vi "SIM Adams manager.vi"(1 "Simulation data":T1={"continuous integrator"=enum."RK 1 (Euler)", "initial time"=0.0, "final time"=6.0, "step size"=0.0, "proposed step size"=0.001, "max step size"=1e-06, "min step size"=0.0, "discrete time step"=0.0, "max step ratio"=3.0, "Diag Eval Stage"=enum."Major Substep", "Substep Index"=0, "Timestep Index"=10.0, "simulation time"=0.0, "current timestep base"=0.1, "proposed step time"=0.0, "absolute tolerance"=0.0, "relative tolerance"=0.0, "step accepted?"=FALSE, "step complete?"=FALSE, "Halt?"=FALSE, "reset integrator?"=FALSE, "machine epsilon"=1.0, "min float"=0.0, "error"={"status"=FALSE, "code"=0, "source"=""}, "Method Order"=0, "Finished Late [i-1]"=FALSE, "Discrete step?"=FALSE, "NaN and Inf check?"=FALSE, "Final Timestep Index"=0.0, "(maj+disc)or(init)?"=FALSE, "Full Solver Reset"=TRUE, "Execution Mode"=enum."Simulate to Completion", "check vector sizes?"=FALSE, "solver handles zc?"=FALSE, "Simulation Registry"={"Current Idx"=0, "Node Tags"=[], "Node Headers"=[], "Node Data"=[], "Cont State data"={"inputs"=[], "outputs"=[], "reset"=[], "lower limits"=[], "upper limits"=[], "limit types"=[], "reset types"=[], "initial conditions"=[], "reset I.C."=[], "limited?"=[], "State Names"=[]}, "DiscreteInfo"={"tick period (sec)"=0.0, "time (ticks)"=0, "fire?"=[], "registry"={"period (sec)"=[], "skew (sec)"=[], "period (tick)"=[], "skew (tick)"=[]}, "discrete \nblocks?"=FALSE, "steps per tick"=0.0, "steps to tick"=0.0, "discrete \ntick?"=FALSE}, "Disc State data"={"Disc States"=[], "State Names"=[]}, "Registry Error"={"Error Block ID"=0, "code"=0}, "ZC Indices"=[]}, "variable step solver?"=FALSE, "First Substep?"=FALSE, "Continuous States?"=FALSE} {"min float" format="%.1e"; "proposed step size" format="%.1e"; "proposed step time" format="%.1e"; "max step ratio" format="%.1e"; "min step size" format="%.1e"; "machine epsilon" format="%.1e"; "discrete time step" format="%.1e"; "max step size" format="%.1e"; "current timestep base" format="%.1e"; "final time" format="%.1e"; "simulation time" format="%.1e"; "relative tolerance" format="%.1e"; "absolute tolerance" format="%.1e"; "Substep Index" format="%.1e"; "step size" format="%.1e"; "initial time" format="%.1e"}) -> (0 "Simulation data out":T1={"continuous integrator"=enum."RK 1 (Euler)", "initial time"=0.0, "final time"=6.0, "step size"=0.0, "proposed step size"=0.001, "max step size"=1e-06, "min step size"=0.0, "discrete time step"=0.0, "max step ratio"=3.0, "Diag Eval Stage"=enum."Major Substep", "Substep Index"=0, "Timestep Index"=10.0, "simulation time"=0.0, "current timestep base"=0.1, "proposed step time"=0.0, "absolute tolerance"=0.0, "relative tolerance"=0.0, "step accepted?"=FALSE, "step complete?"=FALSE, "Halt?"=FALSE, "reset integrator?"=FALSE, "machine epsilon"=1.0, "min float"=0.0, "error"={"status"=FALSE, "code"=0, "source"=""}, "Method Order"=0, "Finished Late [i-1]"=FALSE, "Discrete step?"=FALSE, "NaN and Inf check?"=FALSE, "Final Timestep Index"=0.0, "(maj+disc)or(init)?"=FALSE, "Full Solver Reset"=TRUE, "Execution Mode"=enum."Simulate to Completion", "check vector sizes?"=FALSE, "solver handles zc?"=FALSE, "Simulation Registry"={"Current Idx"=0, "Node Tags"=[], "Node Headers"=[], "Node Data"=[], "Cont State data"={"inputs"=[], "outputs"=[], "reset"=[], "lower limits"=[], "upper limits"=[], "limit types"=[], "reset types"=[], "initial conditions"=[], "reset I.C."=[], "limited?"=[], "State Names"=[]}, "DiscreteInfo"={"tick period (sec)"=0.0, "time (ticks)"=0, "fire?"=[], "registry"={"period (sec)"=[], "skew (sec)"=[], "period (tick)"=[], "skew (tick)"=[]}, "discrete \nblocks?"=FALSE, "steps per tick"=0.0, "steps to tick"=0.0, "discrete \ntick?"=FALSE}, "Disc State data"={"Disc States"=[], "State Names"=[]}, "Registry Error"={"Error Block ID"=0, "code"=0}, "ZC Indices"=[]}, "variable step solver?"=FALSE, "First Substep?"=FALSE, "Continuous States?"=FALSE} {"min float" format="%.1e"; "proposed step size" format="%.1e"; "proposed step time" format="%.1e"; "max step ratio" format="%.1e"; "min step size" format="%.1e"; "machine epsilon" format="%.1e"; "discrete time step" format="%.1e"; "max step size" format="%.1e"; "current timestep base" format="%.1e"; "final time" format="%.1e"; "simulation time" format="%.1e"; "relative tolerance" format="%.1e"; "absolute tolerance" format="%.1e"; "Substep Index" format="%.1e"; "step size" format="%.1e"; "initial time" format="%.1e"})   [LabVIEW 2018]
uses:
  SIM simulation data.ctl
  SIM integration method.ctl
  SIM diagram eval stage.ctl
  SIMSCR Execution Mode.ctl
  SIM Simulation Registry.ctl
  SIM Registry Node Header.ctl
  SIM Registry Node Record.ctl
  SIM trigger type.ctl
  SIM solver state data.ctl
  SIM limit type.ctl
  SIM discrete data.ctl
  SIM Discrete state data.ctl
  SIM Simulation Registry Error.ctl
  SIM Adams stages.ctl
  SIM Adams data.ctl
panel:
  in  "num predictor iterations":i32=1
  in  "Max Order":i32=15
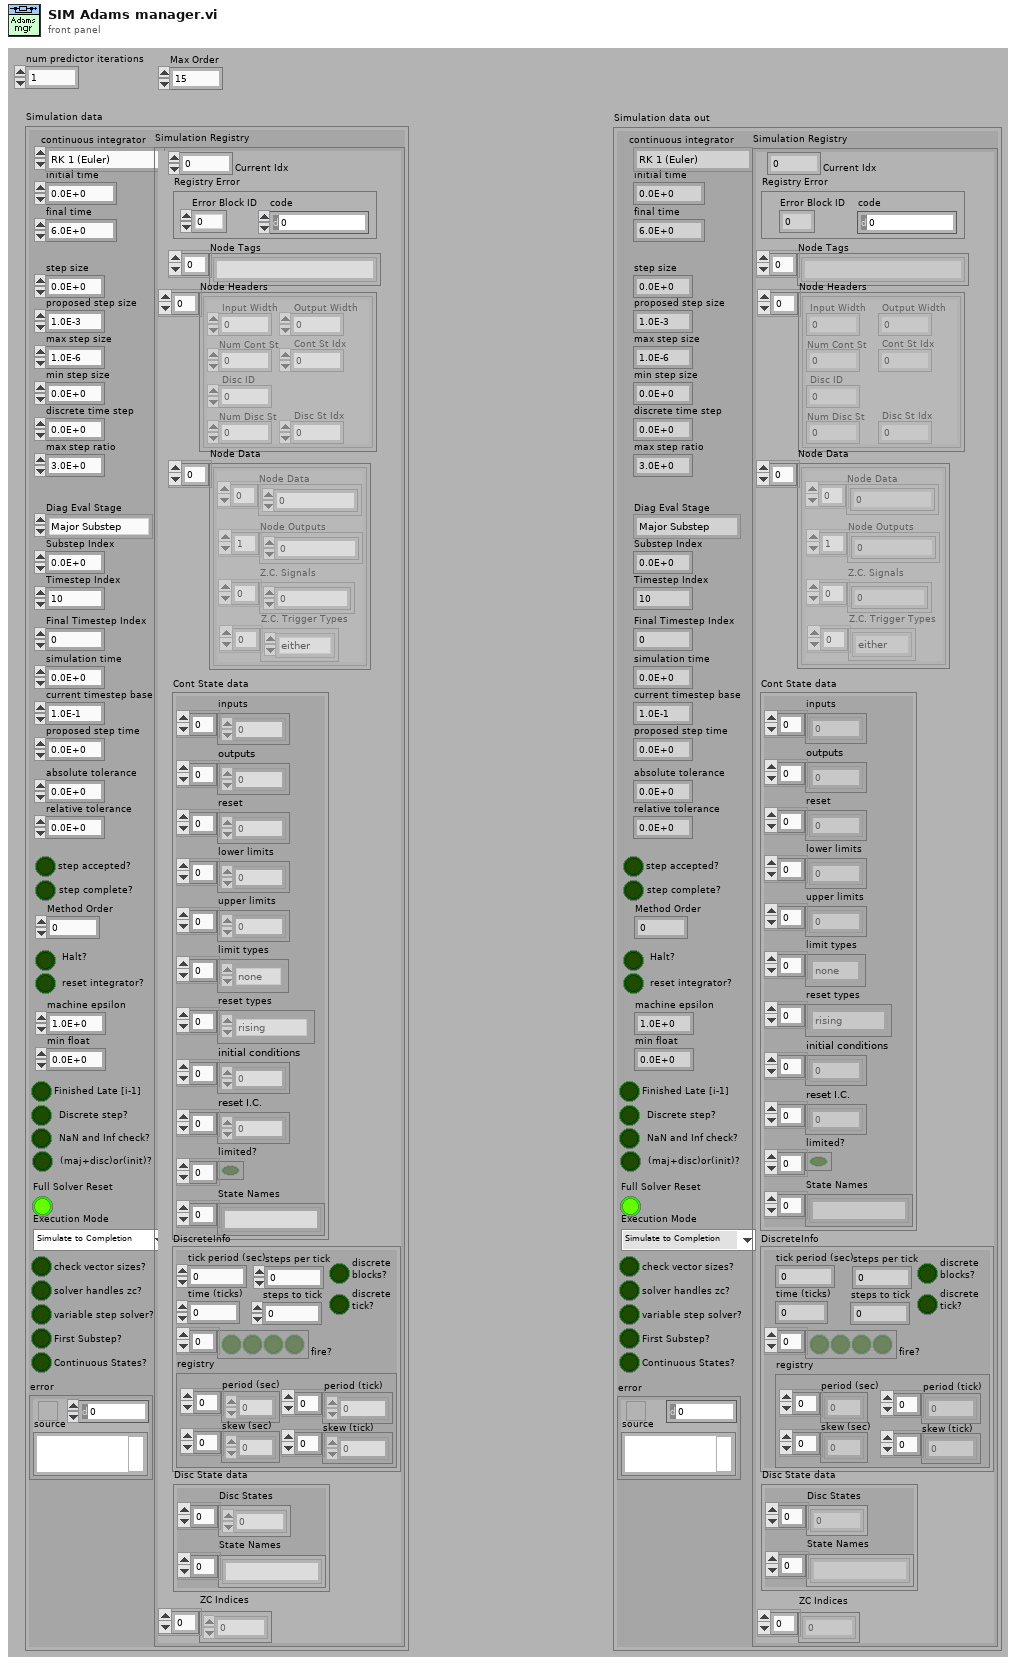
[diagram p1: front panel]
types:
  T1 = typedef "SIM simulation data.ctl" = cluster{"continuous integrator":T2, "initial time":dbl, "final time":dbl, "step size":dbl, "proposed step size":dbl, "max step size":dbl, "min step size":dbl, "discrete time step":dbl, "max step ratio":dbl, "Diag Eval Stage":T3, "Substep Index":i32, "Timestep Index":dbl, "simulation time":dbl, "current timestep base":dbl, "proposed step time":dbl, "absolute tolerance":dbl, "relative tolerance":dbl, "step accepted?":bool, "step complete?":bool, "Halt?":bool, "reset integrator?":bool, "machine epsilon":dbl, "min float":dbl, "error":errorcluster, "Method Order":u32, "Finished Late [i-1]":bool, "Discrete step?":bool, "NaN and Inf check?":bool, "Final Timestep Index":dbl, "(maj+disc)or(init)?":bool, "Full Solver Reset":bool, "Execution Mode":T4, "check vector sizes?":bool, "solver handles zc?":bool, "Simulation Registry":T5, "variable step solver?":bool, "First Substep?":bool, "Continuous States?":bool}
  T2 = typedef "SIM integration method.ctl" = enum16{"RK 1 (Euler)", "Linearizer", "State Query", "Trim Eval", "Adams", "RK 3", "RK 4", "RK 45", "BDF", "RK 2", "RK 23", "Rosenbrock", "Discrete States Only"}
  T3 = typedef "SIM diagram eval stage.ctl" = enum16{"Init", "Minor Substep", "Major Substep", "Final"}
  T4 = typedef "SIMSCR Execution Mode.ctl" = enum16{"Simulate to Completion", "Single Time-Step Simulation (Fixed Step Only)"}
  T5 = typedef "SIM Simulation Registry.ctl" = cluster{"Current Idx":i32, "Node Tags":string[], "Node Headers":T6[], "Node Data":T7[], "Cont State data":T9, "DiscreteInfo":T11, "Disc State data":T12, "Registry Error":T13, "ZC Indices":i32[]}
  T6 = typedef "SIM Registry Node Header.ctl" = cluster{"Input Width":i32, "Disc ID":i32, "Num Cont St":i32, "Cont St Idx":i32, "Num Disc St":i32, "Disc St Idx":i32, "Output Width":i32}
  T7 = typedef "SIM Registry Node Record.ctl" = cluster{"Node Data":dbl[], "Node Outputs":dbl[], "Z.C. Signals":dbl[], "Z.C. Trigger Types":T8[]}
  T8 = typedef "SIM trigger type.ctl" = enum16{"rising", "falling", "either", "none"}
  T9 = typedef "SIM solver state data.ctl" = cluster{"inputs":dbl[], "outputs":dbl[], "reset":dbl[], "lower limits":dbl[], "upper limits":dbl[], "limit types":T10[], "reset types":T8[], "initial conditions":dbl[], "reset I.C.":dbl[], "limited?":bool[], "State Names":string[]}
  T10 = typedef "SIM limit type.ctl" = enum16{"upper", "lower", "both", "none"}
  T11 = typedef "SIM discrete data.ctl" = cluster{"tick period (sec)":dbl, "time (ticks)":i32, "fire?":bool[], "registry":cluster{"period (sec)":dbl[], "skew (sec)":dbl[], "period (tick)":i32[], "skew (tick)":i32[]}, "discrete \nblocks?":bool, "steps per tick":dbl, "steps to tick":dbl, "discrete \ntick?":bool}
  T12 = typedef "SIM Discrete state data.ctl" = cluster{"Disc States":dbl[], "State Names":string[]}
  T13 = typedef "SIM Simulation Registry Error.ctl" = cluster{"Error Block ID":i32, "code":i32}
  T14 = typedef "SIM Adams stages.ctl" = enum16{"Init", "Predict", "Correct", "Eval Error", "Choose StepSize", "Reset BDFs"}
  T15 = typedef "SIM Adams data.ctl" = cluster{"Adams stage":T14, "AB Coeffs":dbl[], "AM Coeffs":dbl[], "BDFs":dbl[][], "last output":dbl[], "zero array":dbl[], "Current Order":i32, "Max Order":i32, "Steps This Order":i32, "Max Err Order":i32, "#Corrections":i32}
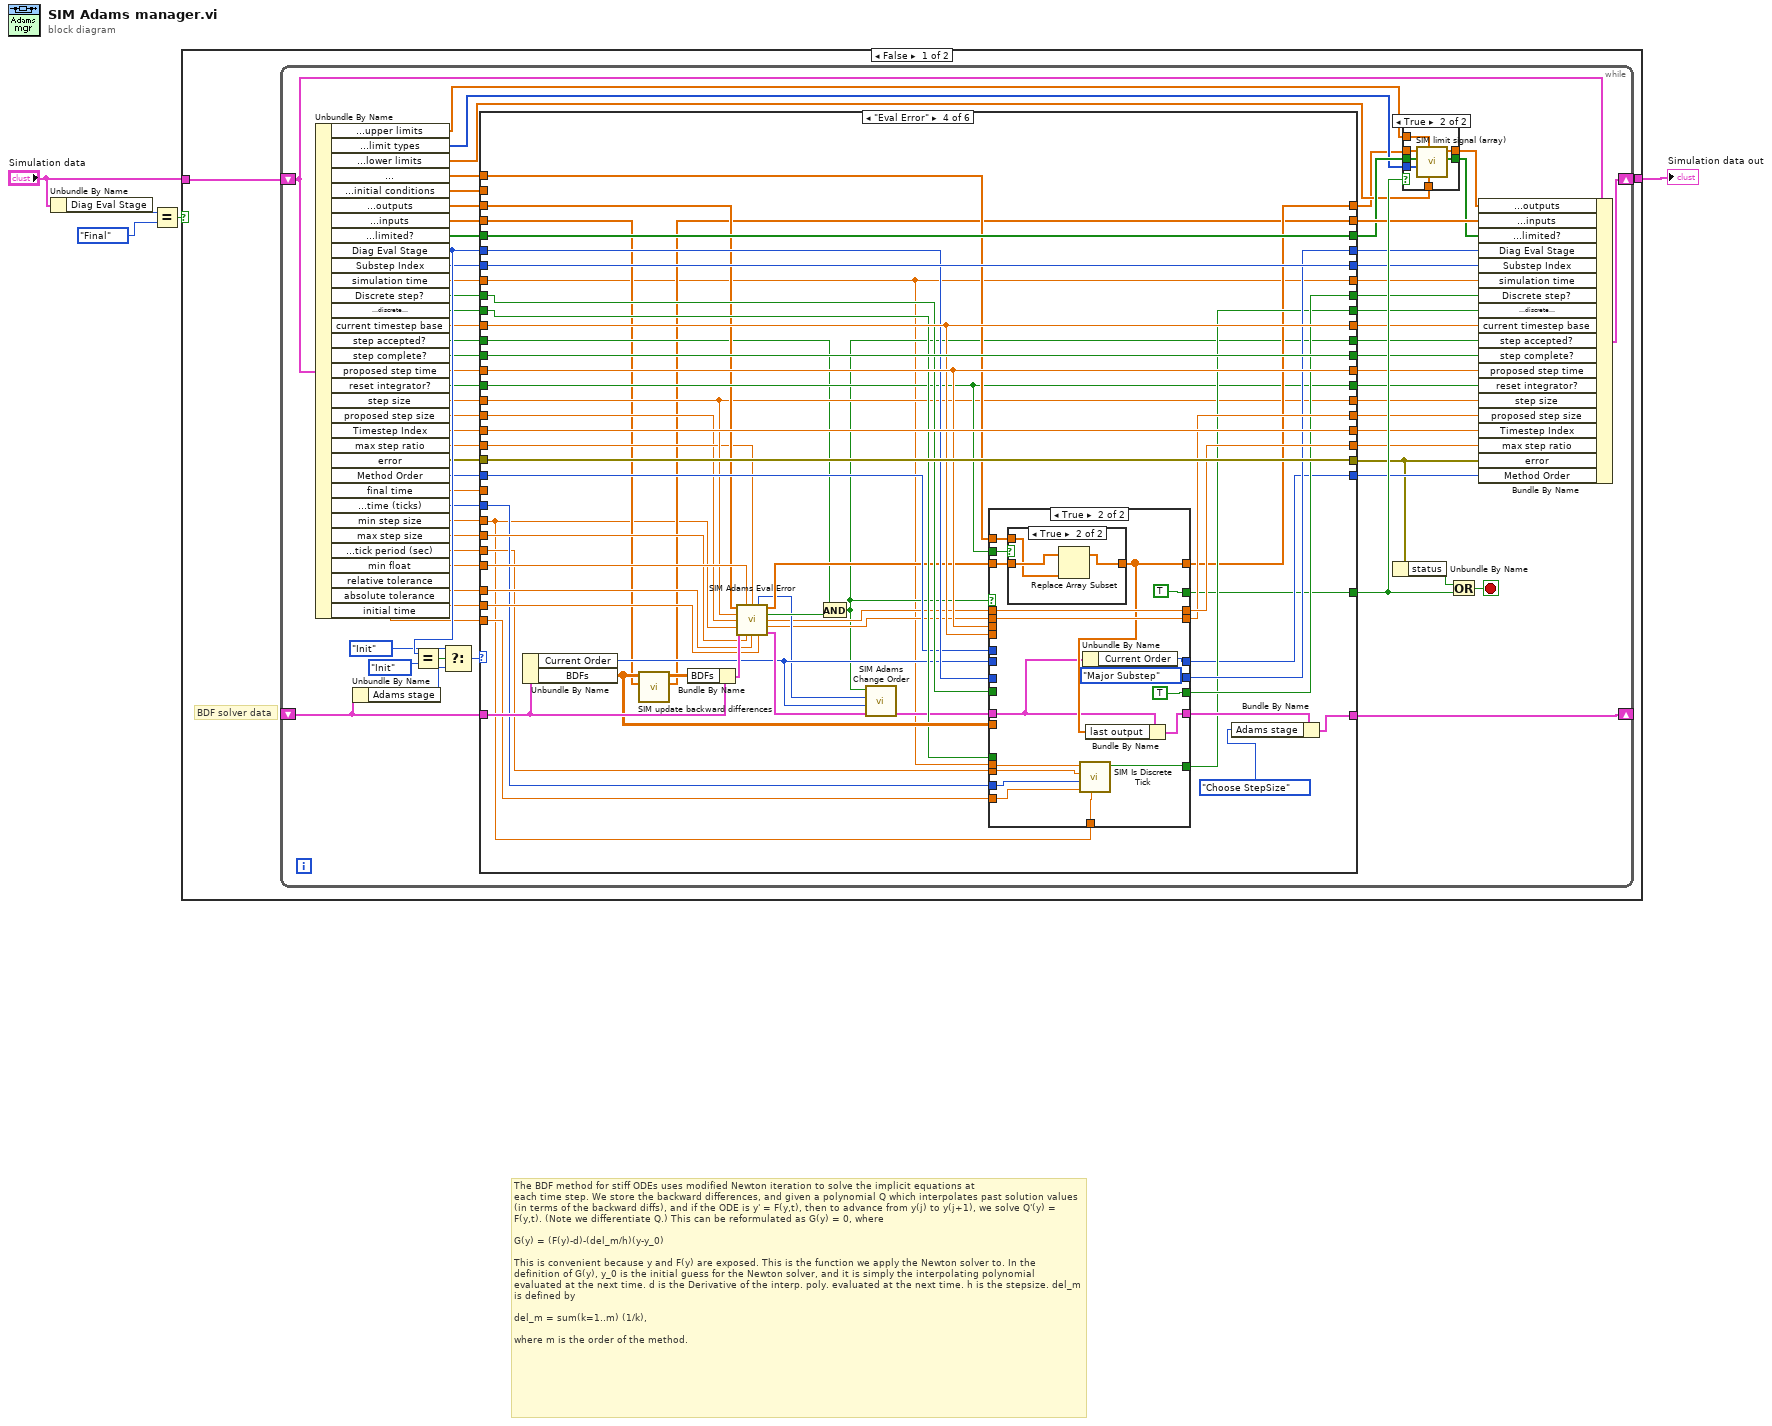
[diagram p0: block diagram]
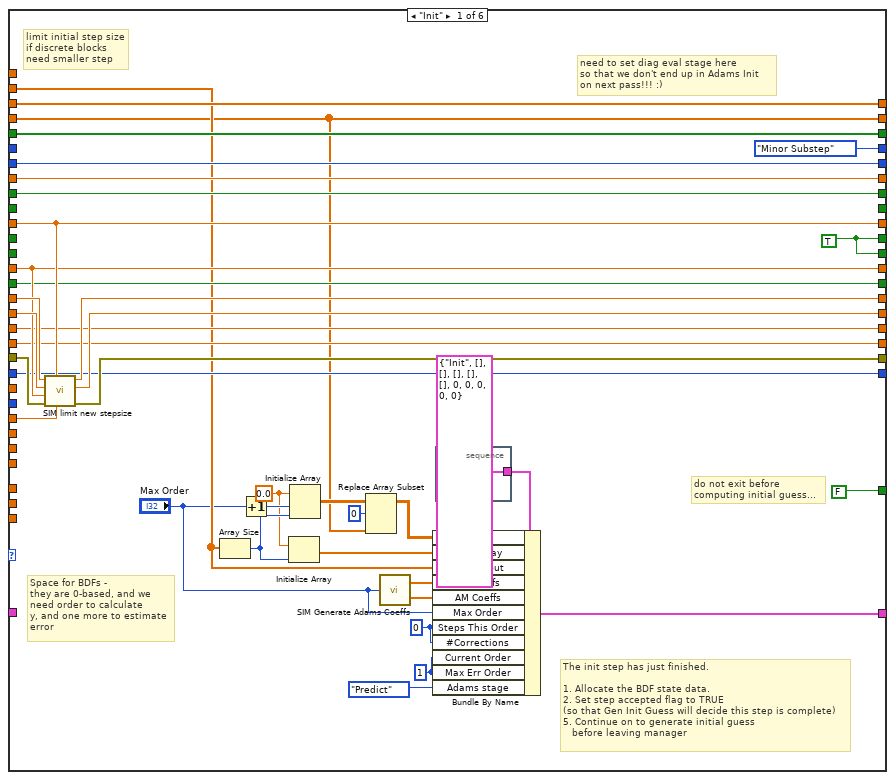
[diagram p3: hidden frame]
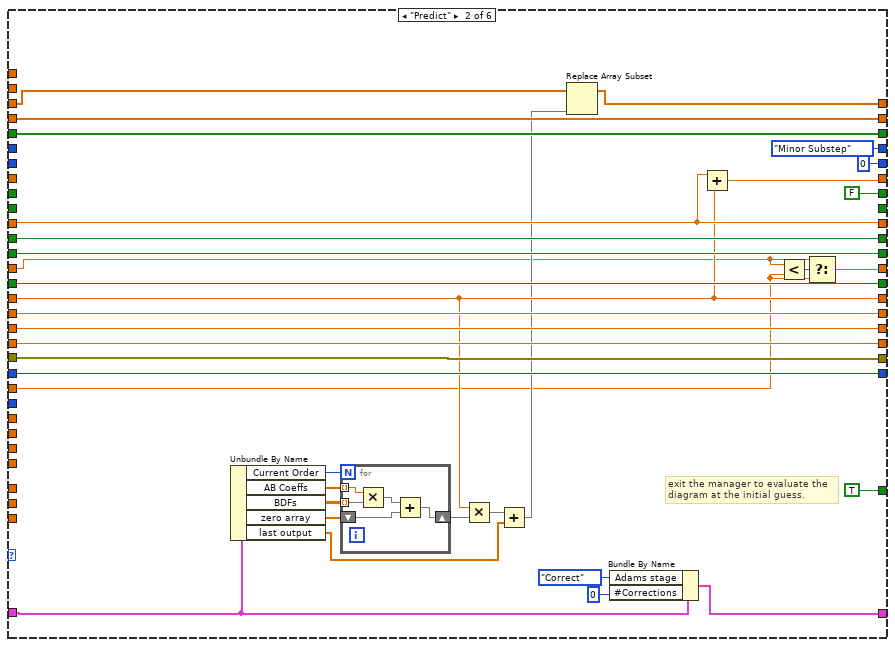
[diagram p4: hidden frame]
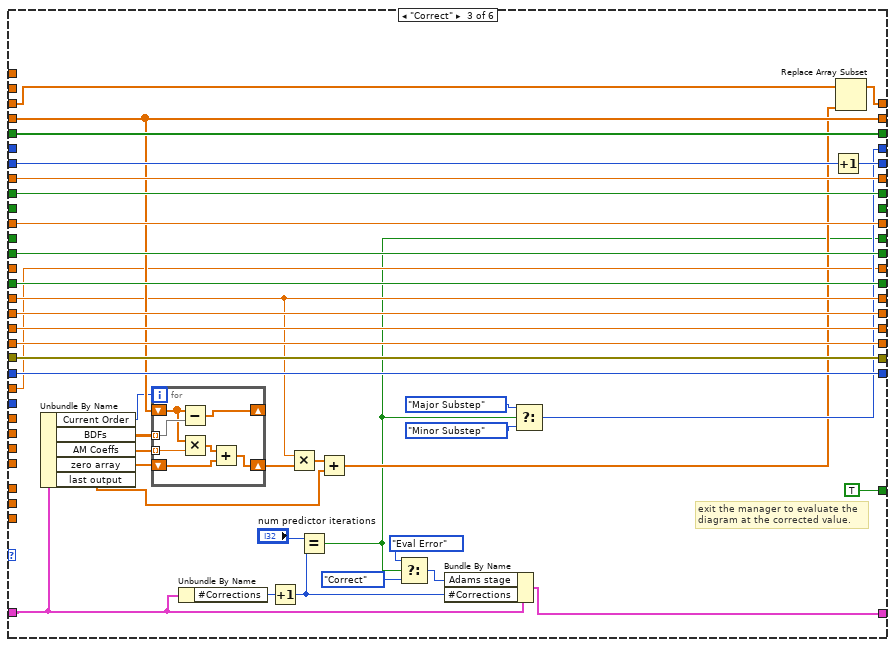
[diagram p5: hidden frame]
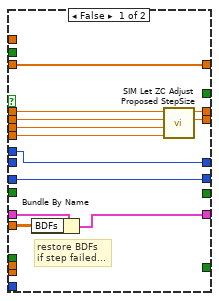
[diagram p6: hidden frame]
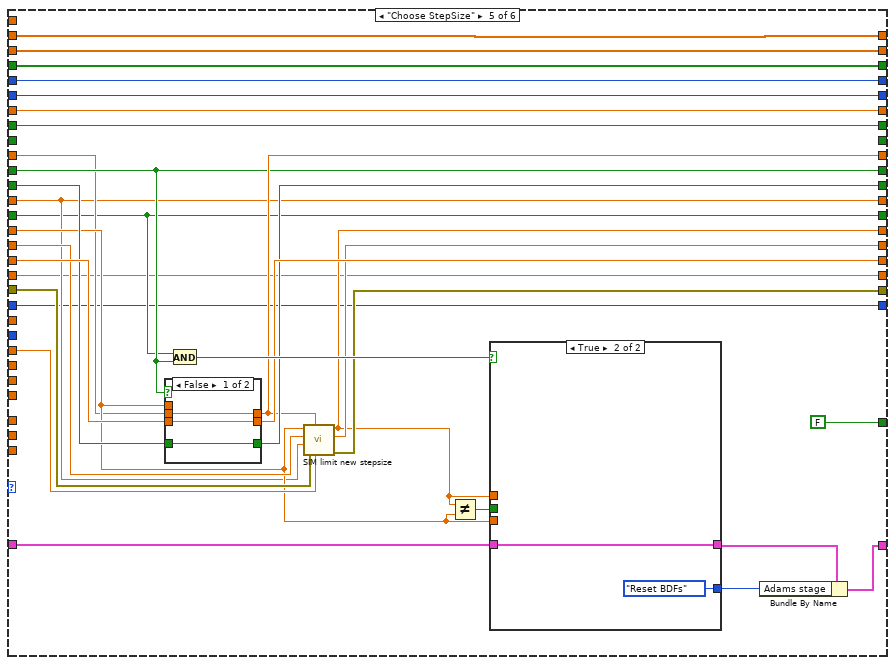
[diagram p8: hidden frame]
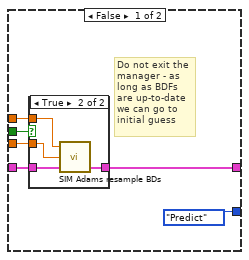
[diagram p9: hidden frame]
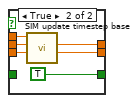
[diagram p11: hidden frame]
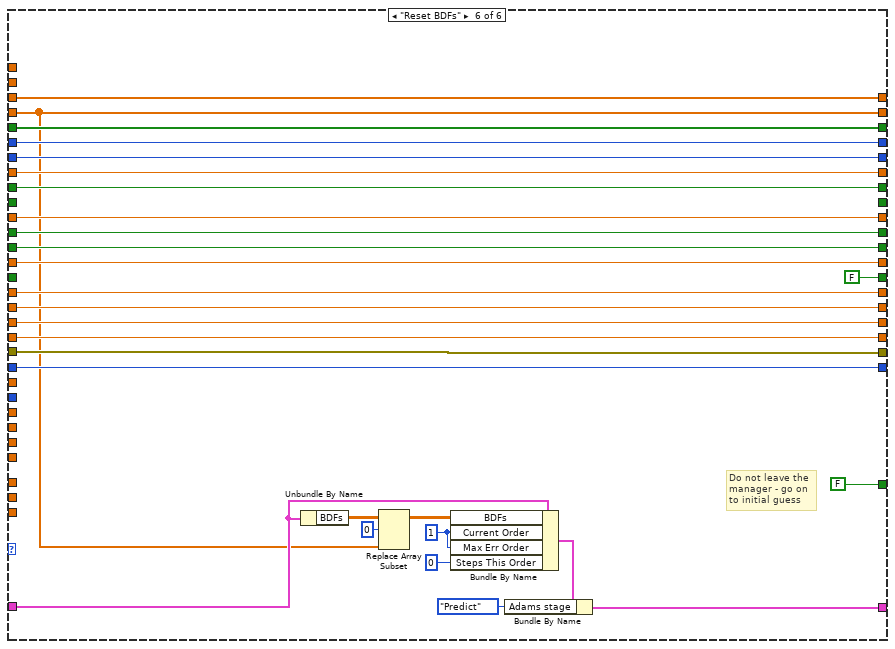
[diagram p12: hidden frame]
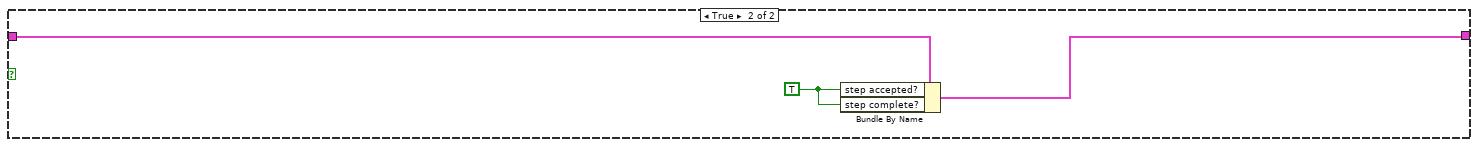
[diagram p13: hidden frame]
diagram:
  # "The BDF method for stiff ODEs uses modified Newton iteration to solve the implicit equations at\neach time step. We store the backward differences, and given a polynomial Q which interpolates past solution values (in terms of the backward diffs), and if the ODE is y' = F(y,t), then to advance from y(j) to y(j+1), we solve Q'(y) = F(y,t). (Note we differentiate Q.) This can be reformulated as G(y) = 0, where \n\nG(y) = (F(y)-d)-(del_m/h)(y-y_0)\n\nThis is convenient because y and F(y) are exposed. This is the function we apply the Newton solver to. In the definition of G(y), y_0 is the initial guess for the Newton solver, and it is simply the interpolating polynomial evaluated at the next time. d is the Derivative of the interp. poly. evaluated at the next time. h is the stepsize. del_m is defined by\n\ndel_m = sum(k=1..m) (1/k),\n\nwhere m is the order of the method."
  n1 = Unbundle By Name("Simulation data") -> ("Diag Eval Stage"=w3:T3)
  n2 = Equal?(x=w3, y=SIM_diagram_eval_stage."Final") -> (x = y?=w1:bool)
  n3 = case shown="False" w1 {
    tunnel: [w7 w378] -> w5
    tunnel: "Simulation data" -> [w6 w377]
    frame False {
      # "BDF solver data"
      n4 = while {
        shift-right: [w33] -> w7
        shift-left: w6 -> [w13]
        shift-right: [w11] -> _
        shift-left: _ -> [w70]
        stop <- w71 stop-if-true
        n5 = Unbundle By Name(w13) -> ("Simulation Registry.Cont State data.upper limits"=w16:dbl[], "Simulation Registry.Cont State data.limit types"=w14:T10[], "Simulation Registry.Cont State data.lower limits"=w15:dbl[], "Simulation Registry.Cont State data.reset I.C."=w24:dbl[], "Simulation Registry.Cont State data.initial conditions"=w28:dbl[], "Simulation Registry.Cont State data.outputs"=w37:dbl[], "Simulation Registry.Cont State data.inputs"=w36:dbl[], "Simulation Registry.Cont State data.limited?"=w30:bool[], "Diag Eval Stage"=w65:T3, "Substep Index"=w63:i32, "simulation time"=w61:dbl, "Discrete step?"=w59:bool, "Simulation Registry.DiscreteInfo.discrete \ntick?"=w57:bool, "current timestep base"=w55:dbl, "step accepted?"=w53:bool, "step complete?"=w51:bool, "proposed step time"=w49:dbl, "reset integrator?"=w47:bool, "step size"=w45:dbl, "proposed step size"=w43:dbl, "Timestep Index"=w41:dbl, "max step ratio"=w39:dbl, "error"=w22:errorcluster, "Method Order"=w21:u32, "final time"=w27:dbl, "Simulation Registry.DiscreteInfo.time (ticks)"=w12:i32, "min step size"=w29:dbl, "max step size"=w25:dbl, "Simulation Registry.DiscreteInfo.tick period (sec)"=w34:dbl, "min float"=w26:dbl, "relative tolerance"=w32:dbl, "absolute tolerance"=w31:dbl, "initial time"=w8:dbl)
        n6 = Unbundle By Name(w70) -> ("Adams stage"=w69:T14)
        n7 = Equal?(x=w65, y=SIM_diagram_eval_stage."Init") -> (x = y?=w67:bool)
        n8 = Select(t=SIM_Adams_stages."Init" ("Adams stage"), s=w67, f=w69) -> (s? t:f=w72:T14)
        n9 = case shown="\"Eval Error\"" w72 {
          tunnel: [FALSE TRUE ("finished?") TRUE ("finished?") w238 FALSE FALSE ("finished?")] -> w66
          tunnel: w70 -> [_ w130 w179 w254 w297 w369]
          tunnel: [SIM_diagram_eval_stage."Minor Substep" ("Diag Eval Stage") SIM_diagram_eval_stage."Minor Substep" ("Diag Eval Stage") w167 w246 w309 w367] -> w64
          tunnel: w65 -> [_ _ _ w245 w309 w367]
          tunnel: [w102 0 ("Substep Index") w199 w256 w308 w366] -> w62
          tunnel: w63 -> [w102 _ w200 w256 w308 w366]
          tunnel: w61 -> [w101 _ w198 w212 w307 w365]
          tunnel: [w101 w145 w198 w212 w307 w365] -> w60
          tunnel: [w100 FALSE ("Discrete step?") w197 w244 w306 w364] -> w58
          tunnel: w59 -> [w100 _ w197 w243 w306 w364]
          tunnel: w57 -> [_ _ _ w241 _ _]
          tunnel: [_ _ _ w242 _ _] -> w56
          tunnel: [w99 w146 w196 w247 w312 w363] -> w54
          tunnel: w55 -> [w99 w146 w196 w247 w304 w363]
          tunnel: [w106 w154 w162 w215 w305 w362] -> w52
          tunnel: w53 -> [_ w154 _ w216 w305 w362]
          tunnel: [w106 w153 w195 w260 w320 w361] -> w50
          tunnel: w51 -> [_ w153 w195 w260 w321 w361]
          tunnel: [w98 w122 w166 w248 w303 w360] -> w48
          tunnel: w49 -> [w98 w123 _ w248 w303 w360]
          tunnel: [w97 w152 w194 w235 w302 FALSE ("reset integrator?")] -> w46
          tunnel: w47 -> [w97 w152 w194 w235 w302 _]
          tunnel: [w107 w135 w171 w230 w314 w359] -> w44
          tunnel: w45 -> [w113 w135 w171 w230 w313 w359]
          tunnel: [w109 w151 w188 w249 w316 w358] -> w42
          tunnel: w43 -> [w112 w151 w188 w219 w319 w358]
          tunnel: [w96 w150 w193 w259 w322 w357] -> w40
          tunnel: w41 -> [w96 w150 w193 w259 w323 w357]
          tunnel: [w95 w149 w187 w250 w300 w356] -> w38
          tunnel: w39 -> [w95 w149 w187 w221 w300 w356]
          tunnel: w37 -> [w104 w128 w164 w233 w296 w350]
          tunnel: w36 -> [w83 w155 w178 w214 w311 w349]
          tunnel: [w104 w126 w163 w237 w296 w350] -> w9
          tunnel: [w83 w155 w178 w213 w311 w349] -> w35
          tunnel: w34 -> [_ _ _ w211 _ _]
          tunnel: w32 -> [_ _ _ w228 _ _]
          tunnel: w31 -> [_ _ _ w227 _ _]
          tunnel: w30 -> [w103 w156 w190 w258 w310 w368]
          tunnel: w22 -> [w111 w148 w192 w257 w318 w355]
          tunnel: w29 -> [w110 _ _ w209 w317 _]
          tunnel: [w108 w148 w192 w257 w315 w355] -> w20
          tunnel: w28 -> [w91 _ _ _ _ _]
          tunnel: [w103 w156 w190 w258 w310 w368] -> w17
          tunnel: w27 -> [_ w124 w166 _ _ _]
          tunnel: w26 -> [_ _ _ w234 _ _]
          tunnel: w25 -> [_ _ _ w229 _ _]
          tunnel: w24 -> [_ _ _ w236 _ _]
          tunnel: [w94 w147 w191 w239 w301 w354] -> w23
          tunnel: w21 -> [w94 w147 w191 w240 w301 w354]
          tunnel: w12 -> [_ _ _ w217 _ _]
          tunnel: [w84 w129 w181 w253 w298 w351] -> w11
          tunnel: w8 -> [_ _ _ w210 _ _]
          frame "Init" {
            w85 = 0 ("Steps This Order")
            w87 = 1 ("Max Order")
            w106 = TRUE ("step complete?")
            w116 = 0.0
            # "need to set diag eval stage here\nso that we don't end up in Adams Init\non next pass!!! :)"
            # "limit initial step size\nif discrete blocks\nneed smaller step"
            # "do not exit before\ncomputing initial guess..."
            # "The init step has just finished.\n\n1. Allocate the BDF state data.\n2. Set step accepted flag to TRUE\n(so that Gen Init Guess will decide this step is complete)\n5. Continue on to generate initial guess\n   before leaving manager"
            # "Space for BDFs - \nthey are 0-based, and we\nneed order to calculate\ny, and one more to estimate\nerror"
            n10 = call "SIM limit new stepsize.vi"("min step size"=w110, "current timestep base"=w99, "error"=w111, "proposed step time"=w98, "proposed step size"=w112, "step size"=w113) -> ("error out"=w108:errorcluster, "proposed step size"=w109:dbl, "step size"=w107:dbl)  [unwired: 3 out]
            n11 = Array Size(array=w91) -> (size(s)=w117:i32)
            n12 = Increment(x="Max Order") -> (x+1=w119:i32)
            n13 = Initialize Array(w116, w117) -> (w92:dbl[])
            n14 = Initialize Array(w116, w119, w117) -> (w114:dbl[][])
            n15 = Replace Array Subset(array=w114, new element=w83, index (row)=0) -> (w118:dbl[][])  [unwired: 1 in]
            n16 = call "SIM Generate Adams Coeffs.vi"("Max Order"="Max Order") -> ("AB Coefficients"=w90:dbl[], "AM Coefficients"=w89:dbl[])
            n17 = stacked-sequence {
              tunnel: [T15 {"Adams stage"=enum."Init", "AB Coeffs"=[], "AM Coeffs"=[], "BDFs"=[], "last output"=[], "zero array"=[], "Current Order"=0, "Max Order"=0, "Steps This Order"=0, "Max Err Order"=0, "#Corrections"=0} ("BDF data")] -> w93
              frame #0 {
              }
            }
            n18 = Bundle By Name(cluster=w93, "BDFs"=w118, "zero array"=w92, "last output"=w91, "AB Coeffs"=w90, "AM Coeffs"=w89, "Max Order"="Max Order", "Steps This Order"=w85, "#Corrections"=w85, "Current Order"=w87, "Max Err Order"=w87, "Adams stage"=SIM_Adams_stages."Predict" ("Enum")) -> (w84:T15)
          }
          frame "Predict" {
            # "exit the manager to evaluate the \ndiagram at the initial guess."
            n19 = Unbundle By Name(w130) -> ("Current Order"=w139:i32, "AB Coeffs"=w138:dbl[], "BDFs"=w142:dbl[][], "zero array"=w141:dbl[], "last output"=w136:dbl[])
            n20 = for {
              N: w139 -> [_]
              shift-right: [w160] -> w140
              shift-left: w141 -> [w161]
              tunnel: w142 -> [w159] mode=indexing
              tunnel: w138 -> [w157] mode=indexing
              n21 = Multiply(x=w157, y=w159) -> (x*y=w158:dbl[])
              n22 = Add(x=w158, y=w161) -> (x+y=w160:dbl[])
            }
            n23 = Multiply(x=w135, y=w140) -> (x*y=w137:dbl[])
            n24 = Add(x=w137, y=w136) -> (x+y=w127:dbl[])
            n25 = Replace Array Subset(array=w128, new element=w127) -> (w126:dbl[])  [unwired: 1 in]
            n26 = Bundle By Name(cluster=w130, "Adams stage"=SIM_Adams_stages."Correct", "#Corrections"=0) -> (w129:T15)
            n27 = Add(x=w146, y=w135) -> (x+y=w145:dbl)
            n28 = Less?(x=w123, y=w124) -> (x < y?=w125:bool)
            n29 = Select(t=w123, s=w125, f=w124) -> (s? t:f=w122:dbl)
          }
          frame "Correct" {
            # "exit the manager to evaluate the \ndiagram at the corrected value."
            n30 = Unbundle By Name(w179) -> ("Current Order"=w176:i32, "BDFs"=w177:dbl[][], "AM Coeffs"=w175:dbl[], "zero array"=w174:dbl[], "last output"=w170:dbl[])
            n31 = for {
              N: w176 -> [_]
              shift-right: [w206] -> w172
              shift-left: w174 -> [w207]
              tunnel: w175 -> [w205] mode=indexing
              tunnel: w177 -> [w203] mode=indexing
              shift-right: [w202] -> _
              shift-left: w178 -> [w201]
              n32 = Subtract(x=w201, y=w203) -> (x-y=w202:dbl[])
              n33 = Multiply(x=w201, y=w205) -> (x*y=w204:dbl[])
              n34 = Add(x=w204, y=w207) -> (x+y=w206:dbl[])
            }
            n35 = Unbundle By Name(w179) -> ("#Corrections"=w186:i32)
            n36 = Increment(x=w186) -> (x+1=w185:i32)
            n37 = Multiply(x=w171, y=w172) -> (x*y=w173:dbl[])
            n38 = Equal?(x="num predictor iterations", y=w185) -> (x = y?=w162:bool)
            n39 = Add(x=w173, y=w170) -> (x+y=w165:dbl[])
            n40 = Select(t=SIM_Adams_stages."Eval Error", s=w162, f=SIM_Adams_stages."Correct" ("Adams stage")) -> (s? t:f=w182:T14)
            n41 = Bundle By Name(cluster=w179, "Adams stage"=w182, "#Corrections"=w185) -> (w181:T15)
            n42 = Select(t=SIM_diagram_eval_stage."Major Substep", s=w162, f=SIM_diagram_eval_stage."Minor Substep" ("Diagram Eval Stage")) -> (s? t:f=w167:T3)
            n43 = Increment(x=w200) -> (x+1=w199:i32)
            n44 = Replace Array Subset(array=w164, new element=w165) -> (w163:dbl[])  [unwired: 1 in]
          }
          frame "Eval Error" {
            n45 = Unbundle By Name(w254) -> ("Current Order"=w223:i32, "BDFs"=w251:dbl[][])
            n46 = call "SIM update backward differences.vi"("New y"=w214, "Backward differences"=w251) -> ("New y out"=w213:dbl[], "New Backward differences"=w255:dbl[][])  [unwired: 8 out]
            n47 = Bundle By Name(cluster=w254, "BDFs"=w255) -> (w231:T15)
            n48 = call "SIM Adams Eval Error.vi"("outputs"=w233, "min float"=w234, "max step ratio"=w221, "step size"=w230, "proposed step size"=w219, "min step size"=w209, "Adams data"=w231, "max step size"=w229, "relative tolerance"=w228, "absolute tolerance"=w227) -> ("proposed new order out"=w222:i32, "outputs out"=w232:dbl[], "step accepted? out"=w226:bool, "proposed max step ratio out"=w220:dbl, "proposed step size out"=w218:dbl, "Adams data out"=w225:T15)
            n49 = And(x=w216, y=w226) -> (x .and. y?=w215:bool)
            n50 = call "SIM Adams Change Order.vi"("Adams data"=w225, "Current Order"=w223, "proposed new order"=w222, "Step Accepted?"=w215) -> ("Adams data out"=w224:T15)  [unwired: 3 out]
            n51 = case shown="True" w215 {
              tunnel: w251 -> [w272 _]
              tunnel: w224 -> [w271 w280]
              tunnel: [w270 w282] -> w252
              tunnel: w223 -> [_ _]
              tunnel: w235 -> [_ w290]
              tunnel: [_ TRUE] -> w238
              tunnel: w236 -> [_ w288]
              tunnel: [w269 w281] -> w237
              tunnel: w232 -> [w269 w287]
              tunnel: [w262 w279] -> w239
              tunnel: [w261 SIM_diagram_eval_stage."Major Substep" ("Diag Eval Stage")] -> w246
              tunnel: [_ TRUE ("Discrete step?")] -> w244
              tunnel: [w268 w283] -> w250
              tunnel: [w267 w284] -> w249
              tunnel: w220 -> [w266 w283]
              tunnel: w218 -> [w265 w284]
              tunnel: w248 -> [w264 _]
              tunnel: w247 -> [w263 _]
              tunnel: w240 -> [w262 _]
              tunnel: w245 -> [w261 _]
              tunnel: w243 -> [_ _]
              tunnel: w211 -> [_ w277]
              tunnel: w217 -> [_ w276]
              tunnel: [_ w273] -> w242
              tunnel: w241 -> [_ _]
              tunnel: w212 -> [_ w278]
              tunnel: w210 -> [_ w275]
              tunnel: w209 -> [_ w274]
              frame False {
                # "restore BDFs \nif step failed..."
                n52 = Bundle By Name(cluster=w271, "BDFs"=w272) -> (w270:T15)
                n53 = call "SIM Let ZC Adjust Proposed StepSize.vi"("current timestep base"=w263, "proposed step time"=w264, "proposed step size"=w265, "max step ratio"=w266) -> ("proposed step size out"=w267:dbl, "max step ratio out"=w268:dbl)  [unwired: 2 out]
              }
              frame True {
                (unwired) TRUE
                n54 = case shown="True" w290 {
                  tunnel: w288 -> [_ w293]
                  tunnel: [w291 w292] -> w281
                  tunnel: w287 -> [w291 w294]
                  frame False {
                  }
                  frame True {
                    n55 = Replace Array Subset(array=w294, new element=w293) -> (w292:dbl[])  [unwired: 1 in]
                  }
                }
                n56 = call "SIM Is Discrete Tick.vi"("min step size"=w274, "initial time"=w275, "time (ticks)"=w276, "tick period (sec)"=w277, "simulation time"=w278) -> ("Discrete Tick?"=w273:bool)  [unwired: 6 out]
                n57 = Unbundle By Name(w280) -> ("Current Order"=w279:i32)
                n58 = Bundle By Name(cluster=w280, "last output"=w281) -> (w282:T15)
              }
            }
            n59 = Bundle By Name(cluster=w252, "Adams stage"=SIM_Adams_stages."Choose StepSize" ("BDF stage")) -> (w253:T15)
          }
          frame "Choose StepSize" {
            n60 = case shown="False" w305 {
              tunnel: w313 -> [_ w348]
              tunnel: w304 -> [w342 w347]
              tunnel: w323 -> [w341 w346]
              tunnel: [w342 w345] -> w312
              tunnel: [w341 w344] -> w322
              tunnel: [w340 TRUE ("step complete?")] -> w320
              tunnel: w321 -> [w340 _]
              frame False {
              }
              frame True {
                n61 = call "SIM update timestep base.vi"("Timestep Index"=w346, "current timestep base"=w347, "step size"=w348) -> ("Timestep Index out"=w344:dbl, "current timestep base out"=w345:dbl)  [unwired: 3 out]
              }
            }
            n62 = And(x=w302, y=w305) -> (x .and. y?=w324:bool)
            n63 = call "SIM limit new stepsize.vi"("min step size"=w317, "current timestep base"=w312, "error"=w318, "proposed step time"=w303, "proposed step size"=w319, "step size"=w313) -> ("error out"=w315:errorcluster, "proposed step size"=w316:dbl, "step size"=w314:dbl)  [unwired: 3 out]
            n64 = Not Equal?(x=w314, y=w313) -> (x != y?=w326:bool)
            n65 = case shown="True" w324 {
              tunnel: w297 -> [w332 w338]
              tunnel: [w328 w338] -> w325
              tunnel: w313 -> [w331 _]
              tunnel: w314 -> [w330 _]
              tunnel: w326 -> [w329 _]
              tunnel: [SIM_Adams_stages."Predict" ("Adams stage") SIM_Adams_stages."Reset BDFs" ("Adams stage")] -> w299
              frame False {
                # "Do not exit the\nmanager - as \nlong as BDFs\nare up-to-date\nwe can go to\ninitial guess"
                n66 = case shown="True" w329 {
                  tunnel: w332 -> [w333 w337]
                  tunnel: [w333 w336] -> w328
                  tunnel: w331 -> [_ w335]
                  tunnel: w330 -> [_ w334]
                  frame False {
                  }
                  frame True {
                    n67 = call "SIM Adams resample BDs.vi"("Adams data"=w337, "current stepSize"=w335, "new stepSize"=w334) -> ("Adams data out"=w336:T15)  [unwired: 2 out]
                  }
                }
              }
              frame True {
              }
            }
            n68 = Bundle By Name(cluster=w325, "Adams stage"=w299) -> (w298:T15)
          }
          frame "Reset BDFs" {
            w371 = 1 ("Current Order")
            # "Do not leave the\nmanager - go on\nto initial guess"
            n69 = Unbundle By Name(w369) -> ("BDFs"=w374:dbl[][])
            n70 = Replace Array Subset(array=w374, new element=w349, index (row)=0) -> (w372:dbl[][])  [unwired: 1 in]
            n71 = Bundle By Name(cluster=w369, "BDFs"=w372, "Current Order"=w371, "Max Err Order"=w371, "Steps This Order"=0) -> (w376:T15)
            n72 = Bundle By Name(cluster=w376, "Adams stage"=SIM_Adams_stages."Predict") -> (w351:T15)
          }
        }
        n73 = Unbundle By Name(w20) -> ("status"=w68:bool)
        n74 = case shown="True" w66 {
          tunnel: w9 -> [w75 w82]
          tunnel: [w75 w81] -> w19
          tunnel: [w74 w80] -> w18
          tunnel: w17 -> [w74 w79]
          tunnel: w16 -> [_ w78]
          tunnel: w15 -> [_ w77]
          tunnel: w14 -> [_ w76]
          frame False {
          }
          frame True {
            n75 = call "SIM limit signal (array).vi"("lower limits"=w77, "upper limits"=w78, "limit types"=w76, "limited? in"=w79, "inputs"=w82) -> ("limited? out"=w80:bool[], "outputs"=w81:dbl[])  [unwired: 1 in, 4 out]
          }
        }
        n76 = Or(x=w68, y=w66) -> (x .or. y?=w71:bool)
        n77 = Bundle By Name(cluster=w13, "Simulation Registry.Cont State data.outputs"=w19, "Simulation Registry.Cont State data.inputs"=w35, "Simulation Registry.Cont State data.limited?"=w18, "Diag Eval Stage"=w64, "Substep Index"=w62, "simulation time"=w60, "Discrete step?"=w58, "Simulation Registry.DiscreteInfo.discrete \ntick?"=w56, "current timestep base"=w54, "step accepted?"=w52, "step complete?"=w50, "proposed step time"=w48, "reset integrator?"=w46, "step size"=w44, "proposed step size"=w42, "Timestep Index"=w40, "max step ratio"=w38, "error"=w20, "Method Order"=w23) -> (w33:T1)
      }
    }
    frame True {
      w379 = TRUE ("step accepted?")
      n78 = Bundle By Name(cluster=w377, "step accepted?"=w379, "step complete?"=w379) -> (w378:T1)
    }
  }
  "Simulation data out" <- w5
